vi "Teleop.vi"(8 "SwerveDriveDevRef":T1={"DevStatus"={"status"=FALSE, "code"=0, "source"=""}, "TurnMotors[]"=[], "Square Inputs"=FALSE, "Max Output"=1.0, "DriveMotors[]"=[], "WheelOffset[]"=[], "SwerveSensors[]"=[], "RobotSize"={"Width"=[], "Length"=[], "Center"=[]}}, 10 "Match Info":T8={"Autonomous Elapsed Seconds"=0.0, "TeleOp Elapsed Seconds"=0.0, "Disabled Elapsed Seconds"=0.0, "Visited Autonomous"=FALSE, "Visited TeleOp"=FALSE, "Visited Disabled"=FALSE, "Autonomous Settings"={"Autonomous Style"=enum."Independent", "VI Refnum"=refnum}}, 11 "Call Context":T9) -> ()   [LabVIEW 2019]
doc: "This VI is called for each TeleOp packet received from the DS where the robot is not disabled. It is often used to read from the joysticks and update I/O or to update setpoints for timed control loops. It should complete and return within 20 milliseconds or it may miss DS packets."
uses:
  <vilib>/Rock Robotics/WPI/DriverStation/WPI_DriverStationDerivedRobotMode.ctl
  <vilib>/Rock Robotics/WPI/DriverStation/WPI_DriverStationMatch Info.ctl
  <vilib>/Rock Robotics/WPI/ThirdParty/REV Robotics/SPARK MAX/Typedef/Spark MAX Control Type.ctl
  <vilib>/Rock Robotics/WPI/Solenoid/WPI_SolenoidValue.ctl
  <vilib>/Rock Robotics/WPI/Utilities/WPI_GetSetVariantRefNum.vi
  <vilib>/Rock Robotics/Network Tables/NT Write Number.vi
  <vilib>/Rock Robotics/WPI/Solenoid/WPI_SolenoidSetEnum.vi
  New Swerve/Swerve Drive.lvlib
  <vilib>/Rock Robotics/SystemInterfaces/DIO/FPGA_DIOPWMChannel.ctl
  <vilib>/Rock Robotics/WPI/PWM/WPI_PWMDeadband.ctl
  <vilib>/Rock Robotics/WPI/MotorControl/WPI_MotorControlType.ctl
  <vilib>/Rock Robotics/SystemInterfaces/DIO/FPGA_DIOChannel.ctl
  <vilib>/Rock Robotics/WPI/MotorControl/WPI_MotorControlDeviceRef.ctl
  <vilib>/Rock Robotics/SystemInterfaces/AI/FPGA_AIChannel.ctl
  New Swerve/SwerveDriveDevRef.ctl
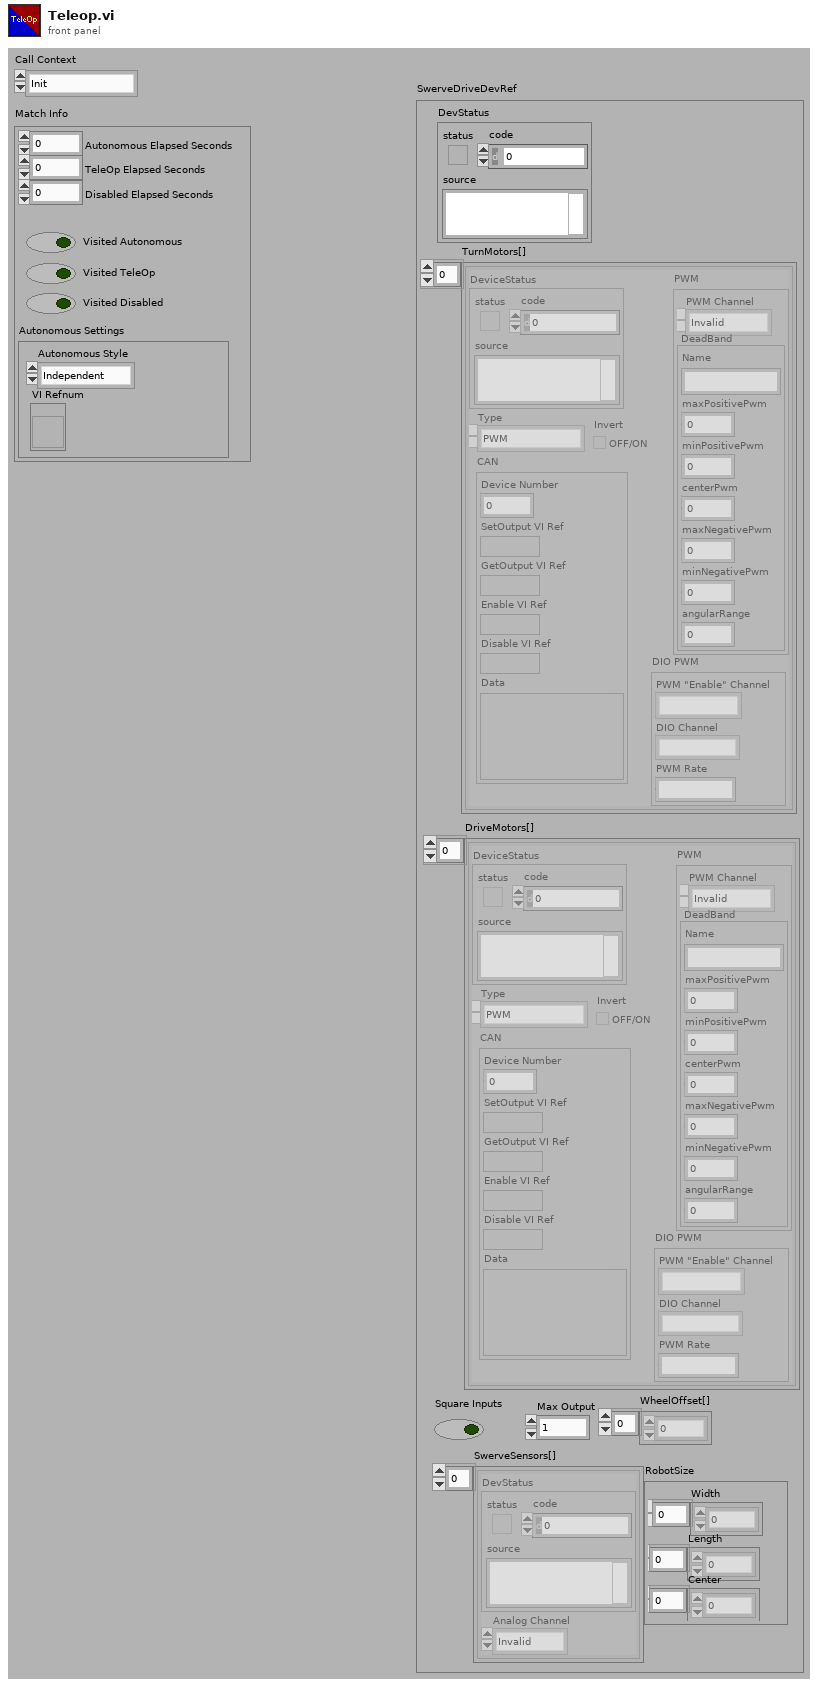
[diagram p1: front panel]
types:
  T1 = typedef "Swerve Drive.lvlib/SwerveDriveDevRef.ctl" = cluster{"DevStatus":errorcluster, "TurnMotors[]":T2[], "Square Inputs":bool, "Max Output":dbl, "DriveMotors[]":T2[], "WheelOffset[]":dbl[], "SwerveSensors[]":cluster{"DevStatus":errorcluster, "Analog Channel":T7}[], "RobotSize":cluster{"Width":dbl[], "Length":dbl[], "Center":dbl[]}}
  T2 = typedef "WPI_MotorControlDeviceRef.ctl" = cluster{"DeviceStatus":errorcluster, "Type":T3, "PWM":cluster{"PWM Channel":T4, "DeadBand":T5}, "CAN":cluster{"Device Number":u8, "SetOutput VI Ref":variant, "GetOutput VI Ref":variant, "Enable VI Ref":variant, "Disable VI Ref":variant, "Data":variant}, "Invert":bool, "DIO PWM":cluster{"PWM \"Enable\" Channel":T4, "DIOChannel":T6, "PWM Rate":dbl}}
  T3 = typedef "WPI_MotorControlType.ctl" = enum16{"PWM", "CAN", "DIO PWM"}
  T4 = typedef "FPGA_DIOPWMChannel.ctl" = enum8{"PWM 0", "PWM 1", "PWM 2", "PWM 3", "PWM 4", "PWM 5", "PWM 6", "PWM 7", "PWM 8", "PWM 9", "PWM MXP 0", "PWM MXP 1", "PWM MXP 2", "PWM MXP 3", "PWM MXP 4", "PWM MXP 5", "PWM MXP 6", "PWM MXP 7", "PWM MXP 8", "PWM MXP 9", "Invalid"}
  T5 = typedef "WPI_PWMDeadband.ctl" = cluster{"Name":string, "maxPositivePwm":i32, "minPositivePwm":i32, "centerPwm":i32, "maxNegativePwm":i32, "minNegativePwm":i32, "angularRange":u16}
  T6 = typedef "FPGA_DIOChannel.ctl" = enum8{"DIO 0", "DIO 1", "DIO 2", "DIO 3", "DIO 4", "DIO 5", "DIO 6", "DIO 7", "DIO 8", "DIO 9", "DIO MXP 0", "DIO MXP 1", "DIO MXP 2", "DIO MXP 3", "DIO MXP 4", "DIO MXP 5", "DIO MXP 6", "DIO MXP 7", "DIO MXP 8", "DIO MXP 9", "DIO MXP 10", "DIO MXP 11", "DIO MXP 12", "DIO MXP 13", "DIO MXP 14", "DIO MXP 15", "SPI Port CS1", "SPI Port CS2", "SPI Port CS3", "SPI Port MISO", "SPI Port MOSI", "Invalid"}
  T7 = typedef "FPGA_AIChannel.ctl" = enum8{"AI 0", "AI 1", "AI 2", "AI 3", "AI MXP 0", "AI MXP 1", "AI MXP 2", "AI MXP 3", "Invalid"}
  T8 = typedef "WPI_DriverStationMatch Info.ctl" = cluster{"Autonomous Elapsed Seconds":dbl, "TeleOp Elapsed Seconds":dbl, "Disabled Elapsed Seconds":dbl, "Visited Autonomous":bool, "Visited TeleOp":bool, "Visited Disabled":bool, "Autonomous Settings":cluster{"Autonomous Style":enum16{"Iterative", "Independent"}, "VI Refnum":refnum<vi>}}
  T9 = typedef "WPI_DriverStationDerivedRobotMode.ctl" = enum16{"Init", "Execute", "Stop"}
  T10 = typedef "WPI_SolenoidValue.ctl" = enum16{"Off", "On", "Forward", "Reverse"}
  T11 = typedef "Spark MAX Control Type.ctl" = enum16{"Percent VBus", "Voltage", "Velocity", "Position", "Smart Motion", "Current", "Smart Velocity"}
  T12 = typedef "WPI_JoystickDevRef.ctl" = cluster{"Device":T13}
  T13 = typedef "WPI_JoystickDeviceEnum.ctl" = enum16{"USB 0", "USB 1", "USB 2", "USB 3", "USB 4", "USB 5"}
  T14 = cluster{"POVs[0]":i16, "POVs[1]":i16, "POVs[2]":i16, "POVs[3]":i16, "POVs[4]":i16, "POVs[5]":i16, "POVs[6]":i16, "POVs[7]":i16, "POVs[8]":i16}
  T15 = cluster{"Axes[0]":dbl, "Axes[1]":dbl, "Axes[2]":dbl, "Axes[3]":dbl, "Axes[4]":dbl, "Axes[5]":dbl, "Axes[6]":dbl, "Axes[7]":dbl, "Axes[8]":dbl}
  T16 = cluster{"Buttons[0]":bool, "Buttons[1]":bool, "Buttons[2]":bool, "Buttons[3]":bool, "Buttons[4]":bool, "Buttons[5]":bool, "Buttons[6]":bool, "Buttons[7]":bool, "Buttons[8]":bool}
  T17 = cluster{"Yaw":dbl, "Roll":dbl, "Pitch":dbl, "Heading":dbl, "Fused Heading":dbl}
  T18 = typedef "WPI_SolenoidDevRef.ctl" = cluster{"DevStatus":errorcluster, "Pneumatics Control Module":u8, "Forward Solenoid Channel":T19, "Reverse Solenoid Channel":T19}
  T19 = typedef "WPI_SolenoidChannel.ctl" = enum8{"Solenoid 0", "Solenoid 1", "Solenoid 2", "Solenoid 3", "Solenoid 4", "Solenoid 5", "Solenoid 6", "Solenoid 7", "Invalid"}
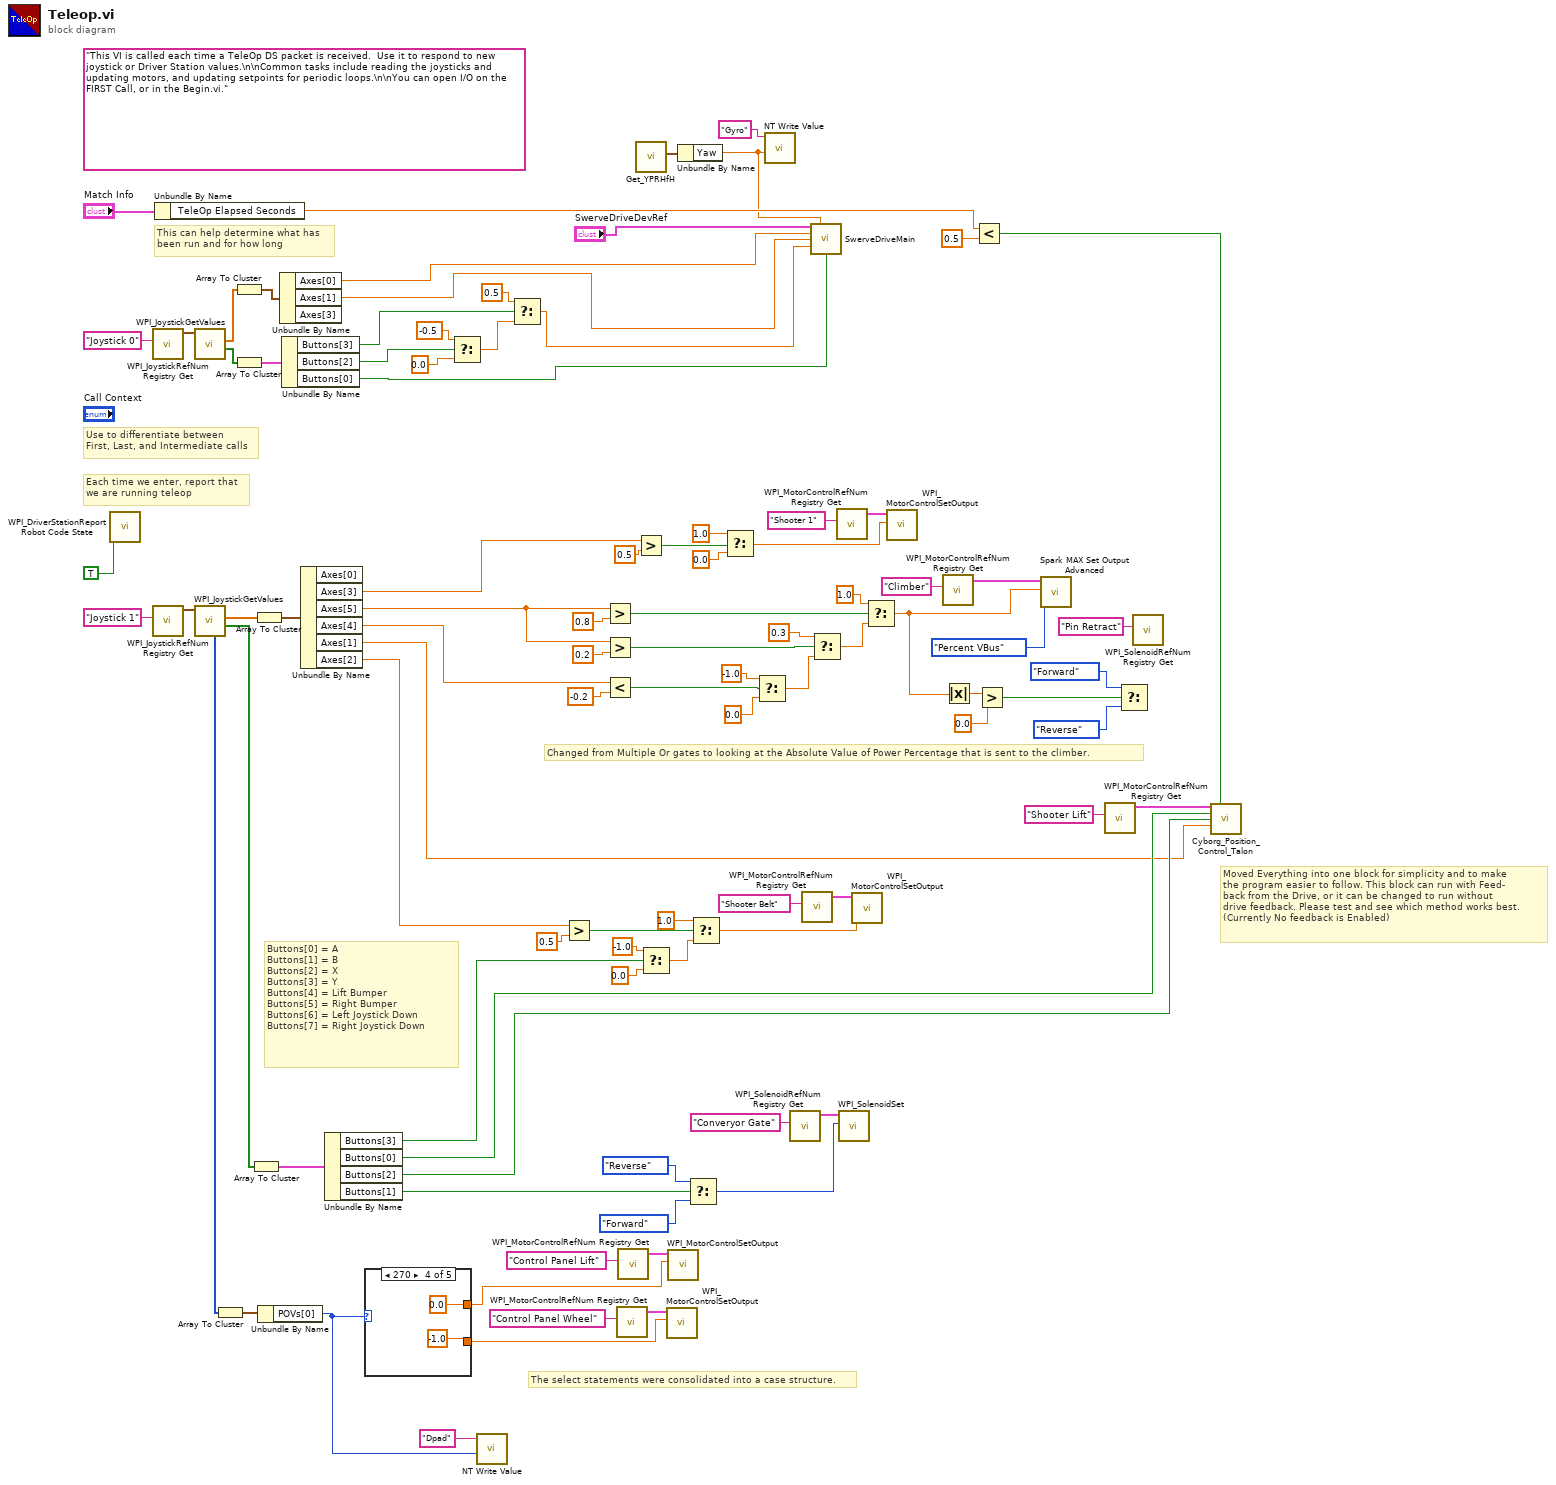
[diagram p0: block diagram]
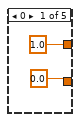
[diagram p2: hidden frame]
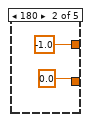
[diagram p3: hidden frame]
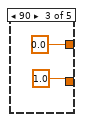
[diagram p4: hidden frame]
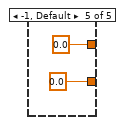
[diagram p5: hidden frame]
diagram:
  (unwired) "This VI is called each time a TeleOp DS packet is received.  Use it to respond to new joystick or Driver Station values.\n\nCommon tasks include reading the joysticks and updating motors, and updating setpoints for periodic loops.\n\nYou can open I/O on the FIRST Call, or in the Begin.vi."
  # "The select statements were consolidated into a case structure."
  # "Moved Everything into one block for simplicity and to make \nthe program easier to follow. This block can run with Feed-\nback from the Drive, or it can be changed to run without \ndrive feedback. Please test and see which method works best.\n(Currently No feedback is Enabled)"
  # "Changed from Multiple Or gates to looking at the Absolute Value of Power Percentage that is sent to the climber."
  # "Buttons[0] = A\nButtons[1] = B\nButtons[2] = X\nButtons[3] = Y\nButtons[4] = Lift Bumper\nButtons[5] = Right Bumper\nButtons[6] = Left Joystick Down\nButtons[7] = Right Joystick Down"
  # "Each time we enter, report that\nwe are running teleop"
  # "Use to differentiate between\nFirst, Last, and Intermediate calls"
  # "This can help determine what has\nbeen run and for how long"
  n1 = call <vilib>:"WPI_DriverStationReport Robot Code State.vi"("TeleOp"=TRUE ("Autonomous")) -> ()  [unwired: 10 in, 1 out]
  n2 = call <vilib>:"WPI_JoystickRefNum Registry Get.vi"("refnum name"="Joystick 0") -> ("JoystickDevRef"=w93:T12)  [unwired: 1 in, 9 out]
  n3 = call <vilib>:"WPI_JoystickRefNum Registry Get.vi"("refnum name"="Joystick 1") -> ("JoystickDevRef"=w77:T12)  [unwired: 1 in, 9 out]
  n4 = Unbundle By Name("Match Info") -> ("TeleOp Elapsed Seconds"=w11:dbl)
  n5 = call <vilib>:"WPI_JoystickGetValues.vi"("JoystickDevRef"=w93) -> ("Buttons"=w88:bool[], "Axes"=w91:dbl[])  [unwired: 6 in, 3 out]
  n6 = call <vilib>:"WPI_JoystickGetValues.vi"("JoystickDevRef"=w77) -> ("Buttons"=w81:bool[], "Axes"=w78:dbl[], "POVs"=w47:i16[])  [unwired: 6 in, 2 out]
  n7 = Array To Cluster(array=w47) -> (cluster=w48:T14)
  n8 = Array To Cluster(array=w91) -> (cluster=w90:T15)
  n9 = Array To Cluster(array=w88) -> (cluster=w89:T16)
  n10 = Array To Cluster(array=w81) -> (cluster=w80:T16)
  n11 = Array To Cluster(array=w78) -> (cluster=w79:T15)
  n12 = Unbundle By Name(w48) -> ("POVs[0]"=w26:i16)
  n13 = Unbundle By Name(w90) -> ("Axes[0]"=w8:dbl, "Axes[1]"=w7:dbl)  [unwired: 1 out]
  n14 = Unbundle By Name(w89) -> ("Buttons[3]"=w83:bool, "Buttons[2]"=w82:bool, "Buttons[0]"=w5:bool)
  n15 = Unbundle By Name(w79) -> ("Axes[3]"=w66:dbl, "Axes[5]"=w18:dbl, "Axes[4]"=w17:dbl, "Axes[1]"=w19:dbl, "Axes[2]"=w12:dbl)  [unwired: 1 out]
  n16 = Unbundle By Name(w80) -> ("Buttons[3]"=w20:bool, "Buttons[0]"=w22:bool, "Buttons[2]"=w21:bool, "Buttons[1]"=w41:bool)
  n17 = case shown="270" w26 {
    tunnel: [1.0 ("t") -1.0 ("t") 0.0 ("t") 0.0 ("t") 0.0 ("t")] -> w25
    tunnel: [0.0 ("f") 0.0 ("f") 1.0 ("f") -1.0 ("f") 0.0 ("f")] -> w24
    frame 0 {
    }
    frame 180 {
    }
    frame 90 {
    }
    frame 270 {
    }
    frame -1, Default {
    }
  }
  n18 = Select(t=-0.5, s=w82, f=0.0) -> (s? t:f=w87:dbl)
  n19 = call-poly <vilib>:"NT Write Value.vi"("Numeric"=w26, "Name"="Dpad") -> ()  [unwired: 9 in, 1 out]
  n20 = Select(t=0.5, s=w83, f=w87) -> (s? t:f=w6:dbl)
  n21 = Greater?(x=w12, y=0.5) -> (0:w70:bool)
  n22 = Greater?(x=w18, y=0.8) -> (0:w27:bool)
  n23 = Greater?(x=w18, y=0.2) -> (0:w28:bool)
  n24 = Less?(x=w17, y=-0.2) -> (x < y?=w29:bool)
  n25 = call <vilib>:"WPI_MotorControlRefNum Registry Get.vi"("refnum name"="Control Panel Wheel") -> ("MotorControlDevRef"=w30:T2)  [unwired: 9 in, 1 out]
  n26 = call <vilib>:"WPI_MotorControlRefNum Registry Get.vi"("refnum name"="Control Panel Lift") -> ("MotorControlDevRef"=w32:T2)  [unwired: 9 in, 1 out]
  n27 = call <vilib>:"Get_YPRHfH.vi"() -> ("YRPHfH"=w4:T17)  [unwired: 11 in]
  n28 = Greater?(x=w66, y=0.5) -> (0:w63:bool)
  n29 = Select(t=-1.0, s=w20, f=0.0) -> (s? t:f=w36:dbl)
  n30 = call <vilib>:"WPI_MotorControlSetOutput.vi"("Output"=w24, "MotorControlDevRef"=w30) -> ()  [unwired: 7 in, 3 out]
  n31 = call <vilib>:"WPI_MotorControlSetOutput.vi"("Output"=w25, "MotorControlDevRef"=w32) -> ()  [unwired: 7 in, 3 out]
  n32 = Unbundle By Name(w4) -> ("Yaw"=w2:dbl)
  n33 = Select(t=WPI_SolenoidValue."Reverse" ("Value"), s=w41, f=WPI_SolenoidValue."Forward" ("Value")) -> (s? t:f=w40:T10)
  n34 = Select(t=1.0, s=w70, f=w36) -> (s? t:f=w71:dbl)
  n35 = Select(t=1.0, s=w63, f=0.0) -> (s? t:f=w62:dbl)
  n36 = Select(t=-1.0, s=w29, f=0.0) -> (s? t:f=w53:dbl)
  n37 = call-poly <vilib>:"NT Write Value.vi"("Numeric"=w2, "Name"="Gyro") -> ()  [unwired: 9 in, 1 out]
  n38 = call <vilib>:"WPI_SolenoidRefNum Registry Get.vi"("refnum name"="Converyor Gate") -> ("SolenoidDevRef"=w45:T18)  [unwired: 9 in, 1 out]
  n39 = call <vilib>:"WPI_MotorControlRefNum Registry Get.vi"("refnum name"="Shooter Belt") -> ("MotorControlDevRef"=w72:T2)  [unwired: 9 in, 1 out]
  n40 = call "SwerveDriveMain.vi"("SwerveDriveDevRef"="SwerveDriveDevRef", "Gyro Angle"=w2, "X"=w8, "Y"=w7, "Z"=w6, "Robot/ Field Centric"=w5) -> ()  [unwired: 8 in, 2 out]
  n41 = Select(t=0.3, s=w28, f=w53) -> (s? t:f=w57:dbl)
  n42 = call <vilib>:"WPI_MotorControlRefNum Registry Get.vi"("refnum name"="Shooter 1") -> ("MotorControlDevRef"=w64:T2)  [unwired: 9 in, 1 out]
  n43 = call-poly <vilib>:"WPI_SolenoidSet.vi"("Value"=w40, "SolenoidDevRef"=w45) -> ()  [unwired: 8 in, 2 out]
  n44 = call <vilib>:"WPI_MotorControlSetOutput.vi"("Output"=w71, "MotorControlDevRef"=w72) -> ()  [unwired: 7 in, 3 out]
  n45 = Select(t=1.0, s=w27, f=w57) -> (s? t:f=w14:dbl)
  n46 = call <vilib>:"WPI_MotorControlSetOutput.vi"("Output"=w62, "MotorControlDevRef"=w64) -> ()  [unwired: 7 in, 3 out]
  n47 = call <vilib>:"WPI_MotorControlRefNum Registry Get.vi"("refnum name"="Climber") -> ("MotorControlDevRef"=w50:T2)  [unwired: 9 in, 1 out]
  n48 = Absolute Value(x=w14) -> (abs(x)=w16:dbl)
  n49 = Less?(x=w11, y=0.5) -> (x < y?=w10:bool)
  n50 = Greater?(x=w16, y=0.0) -> (0:w13:bool)
  n51 = call <vilib>:"Spark MAX Set Output Advanced.vi"("Control Mode"=Spark_MAX_Control_Type."Percent VBus", "Setpoint"=w14, "MotorControlDevRef"=w50) -> ()  [unwired: 7 in, 2 out]
  n52 = call <vilib>:"WPI_MotorControlRefNum Registry Get.vi"("refnum name"="Shooter Lift") -> ("MotorControlDevRef"=w23:T2)  [unwired: 9 in, 1 out]
  n53 = Select(t=WPI_SolenoidValue."Forward" ("Value"), s=w13, f=WPI_SolenoidValue."Reverse" ("Value")) -> ()  [unwired: 1 out]
  n54 = call <vilib>:"WPI_SolenoidRefNum Registry Get.vi"("refnum name"="Pin Retract") -> ()  [unwired: 9 in, 2 out]
  n55 = call "Cyborg_Position_Control_Talon.vi"("PhoenixMotorControlDevRef"=w23, "Drive Feedback"=w10, "Upper"=w22, "Lower"=w21, "Jog Input"=w19) -> ()  [unwired: 11 in]
